vi "Actor Core.vi"(8 "error in":errorcluster, 11 "Panel Form Model in":refnum<class "Panel Form Model.lvclass">) -> (0 "error out":errorcluster, 3 "Actor out":refnum<class "Actor.lvclass">)   [LabVIEW 2020, in "Panel Form Model.lvclass"]
doc: "(<B>Filename</B>: Actor Framework.lvlib:Actor.lvclass:Actor Core.vi)\n\nReceives messages to the actor, reacts to them, and initiates any error handling that may shut the actor down.\n\nDescendant classes may override this VI to append parallel tasks for the actor to complete while it handles messages. Overrides use the Call Parent Class Method node."
uses:
  Panel Form Model.lvclass
  Form Model/Form Model.lvclass
  <vilib>/MGI/Panel Manager/Panel Actor/Panel Actor/Panel Actor.lvclass
  <vilib>/MGI/Panel Manager/Panel Actor/Panel Actor/Launch as Nested Actor.vi
  C:/Users/User/Desktop/Raman Program/Database OOP/forms AF/Form Model/Form Model.lvclass
  C:/Program Files (x86)/National Instruments/LabVIEW 2020/vi.lib/ActorFramework/Actor/Actor.lvclass
  C:/Users/User/Desktop/Raman Program/Database OOP/forms AF/Panel Form Model/Panel Form Model.lvclass
  <vilib>/ActorFramework/Actor/Actor.lvclass
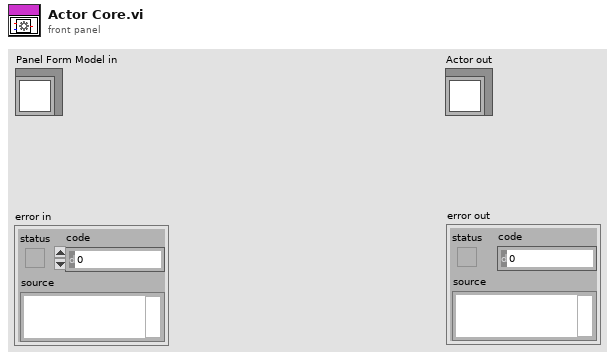
[diagram p1: front panel]
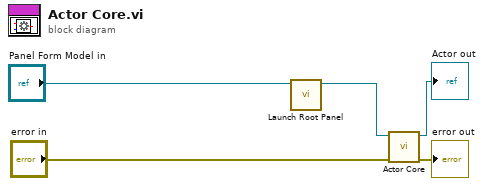
[diagram p0: block diagram]
diagram:
  n1 = call-poly <vilib>:"Launch Root Panel.vi"("Caller Actor in"="Panel Form Model in") -> ("Caller Actor out"=w1:refnum<class "Panel Form Model.lvclass">)  [unwired: 8 in, 2 out]
  n2 = call-parent "Actor Core.vi"("error in"="error in", "Form Model in"=w1) -> ("error out"=→"error out":errorcluster, "Actor out"=→"Actor out":refnum<class "Actor.lvclass">)  [unwired: 8 in]
